vi "Measurement.vi"(8 "error in (no error)":errorcluster, 11 "IV in":refnum<class "IV.lvclass">) -> (0 "error out":errorcluster, 1 "Finish?":bool, 2 "Result":dbl, 3 "IV out":refnum<class "IV.lvclass">)   [LabVIEW 2014, in "IV.lvclass"]
uses:
  IV.lvclass
  meas/IV_meas.lvclass
  data/IV_data.lvclass
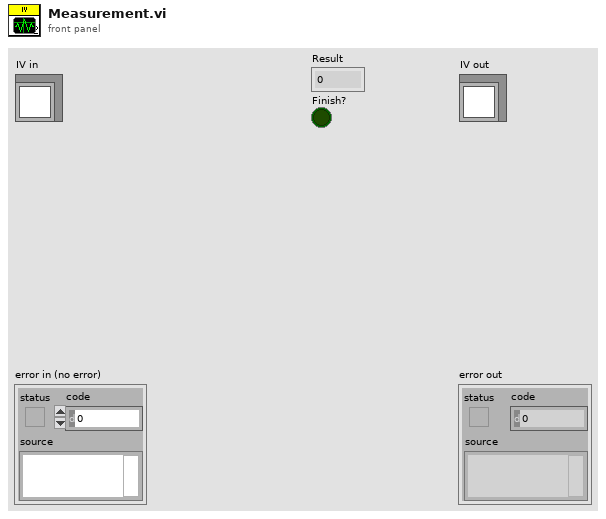
[diagram p1: front panel]
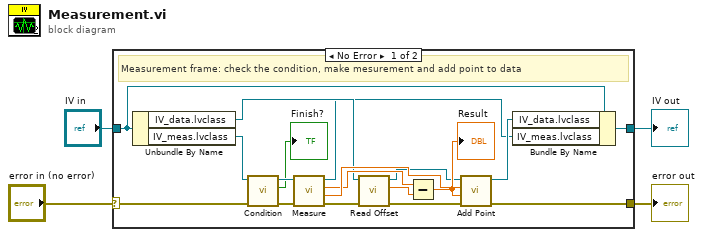
[diagram p0: block diagram]
diagram:
  n1 = case shown="No Error" "error in (no error)" {
    selector: "error in (no error)" -> [w16 w24]
    tunnel: "IV in" -> [w8 w23]
    tunnel: [w5 w23] -> w2
    tunnel: [w9 w24] -> w1
    frame No Error {
      # "Measurement frame: check the condition, make mesurement and add point to data"
      n2 = Unbundle By Name(w8) -> ("IV_data.lvclass"=w14:refnum<class "IV_data.lvclass">, "IV_meas.lvclass"=w19:refnum<class "IV_meas.lvclass">)
      n3 = call "Condition.vi"("error in (no error)"=w16, "IV_meas in"=w19) -> ("error out"=w15:errorcluster, "Finish?"=→"Finish?":bool, "IV_meas out"=w18:refnum<class "IV_meas.lvclass">)  [unwired: 7 in]
      n4 = call-dynamic "Measure.vi"("error in (no error)"=w15, "IV_meas in"=w18) -> ("error out"=w11:errorcluster, "Current Value"=w22:dbl, "Result"=w20:dbl, "IV_meas out"=w6:refnum<class "IV_meas.lvclass">)  [unwired: 6 in]
      n5 = call "Read Offset.vi"("error in (no error)"=w11, "IV_data in"=w14) -> ("error out"=w10:errorcluster, "Offset"=w13:dbl, "IV_data out"=w12:refnum<class "IV_data.lvclass">)  [unwired: 7 in]
      n6 = Subtract(x=w20, y=w13) -> (x-y=w21:dbl)
      "Result" <- w21
      n7 = call-dynamic "Add Point.vi"("error in (no error)"=w10, "Y"=w21, "X"=w22, "IV_data in"=w12) -> ("error out"=w9:errorcluster, "IV_data out"=w7:refnum<class "IV_data.lvclass">)  [unwired: 6 in]
      n8 = Bundle By Name(cluster=w8, "IV_data.lvclass"=w7, "IV_meas.lvclass"=w6) -> (w5:refnum<class "IV.lvclass">)
    }
    frame Error {
    }
  }
  "error out" <- w1
  "IV out" <- w2
